vi "Client_Progetto.vi"() -> ()   [LabVIEW 2023]
uses:
  <vilib>/measure/madcrms.llb/Basic Averaged DC-RMS for 1 Chan.vi
  <vilib>/measure/NI_MAPro.lvlib
panel:
  out "Elettromiogramma (EMG)":waveform(dbl)[](graph)
  out "Valore minimo":dbl format="%0.2f"
  out "Valore massimo":dbl format="%0.2f"
  out "Valore efficace (RMS)":dbl format="%0.2p"
  out "error out":errorcluster
  out "error out 2":errorcluster
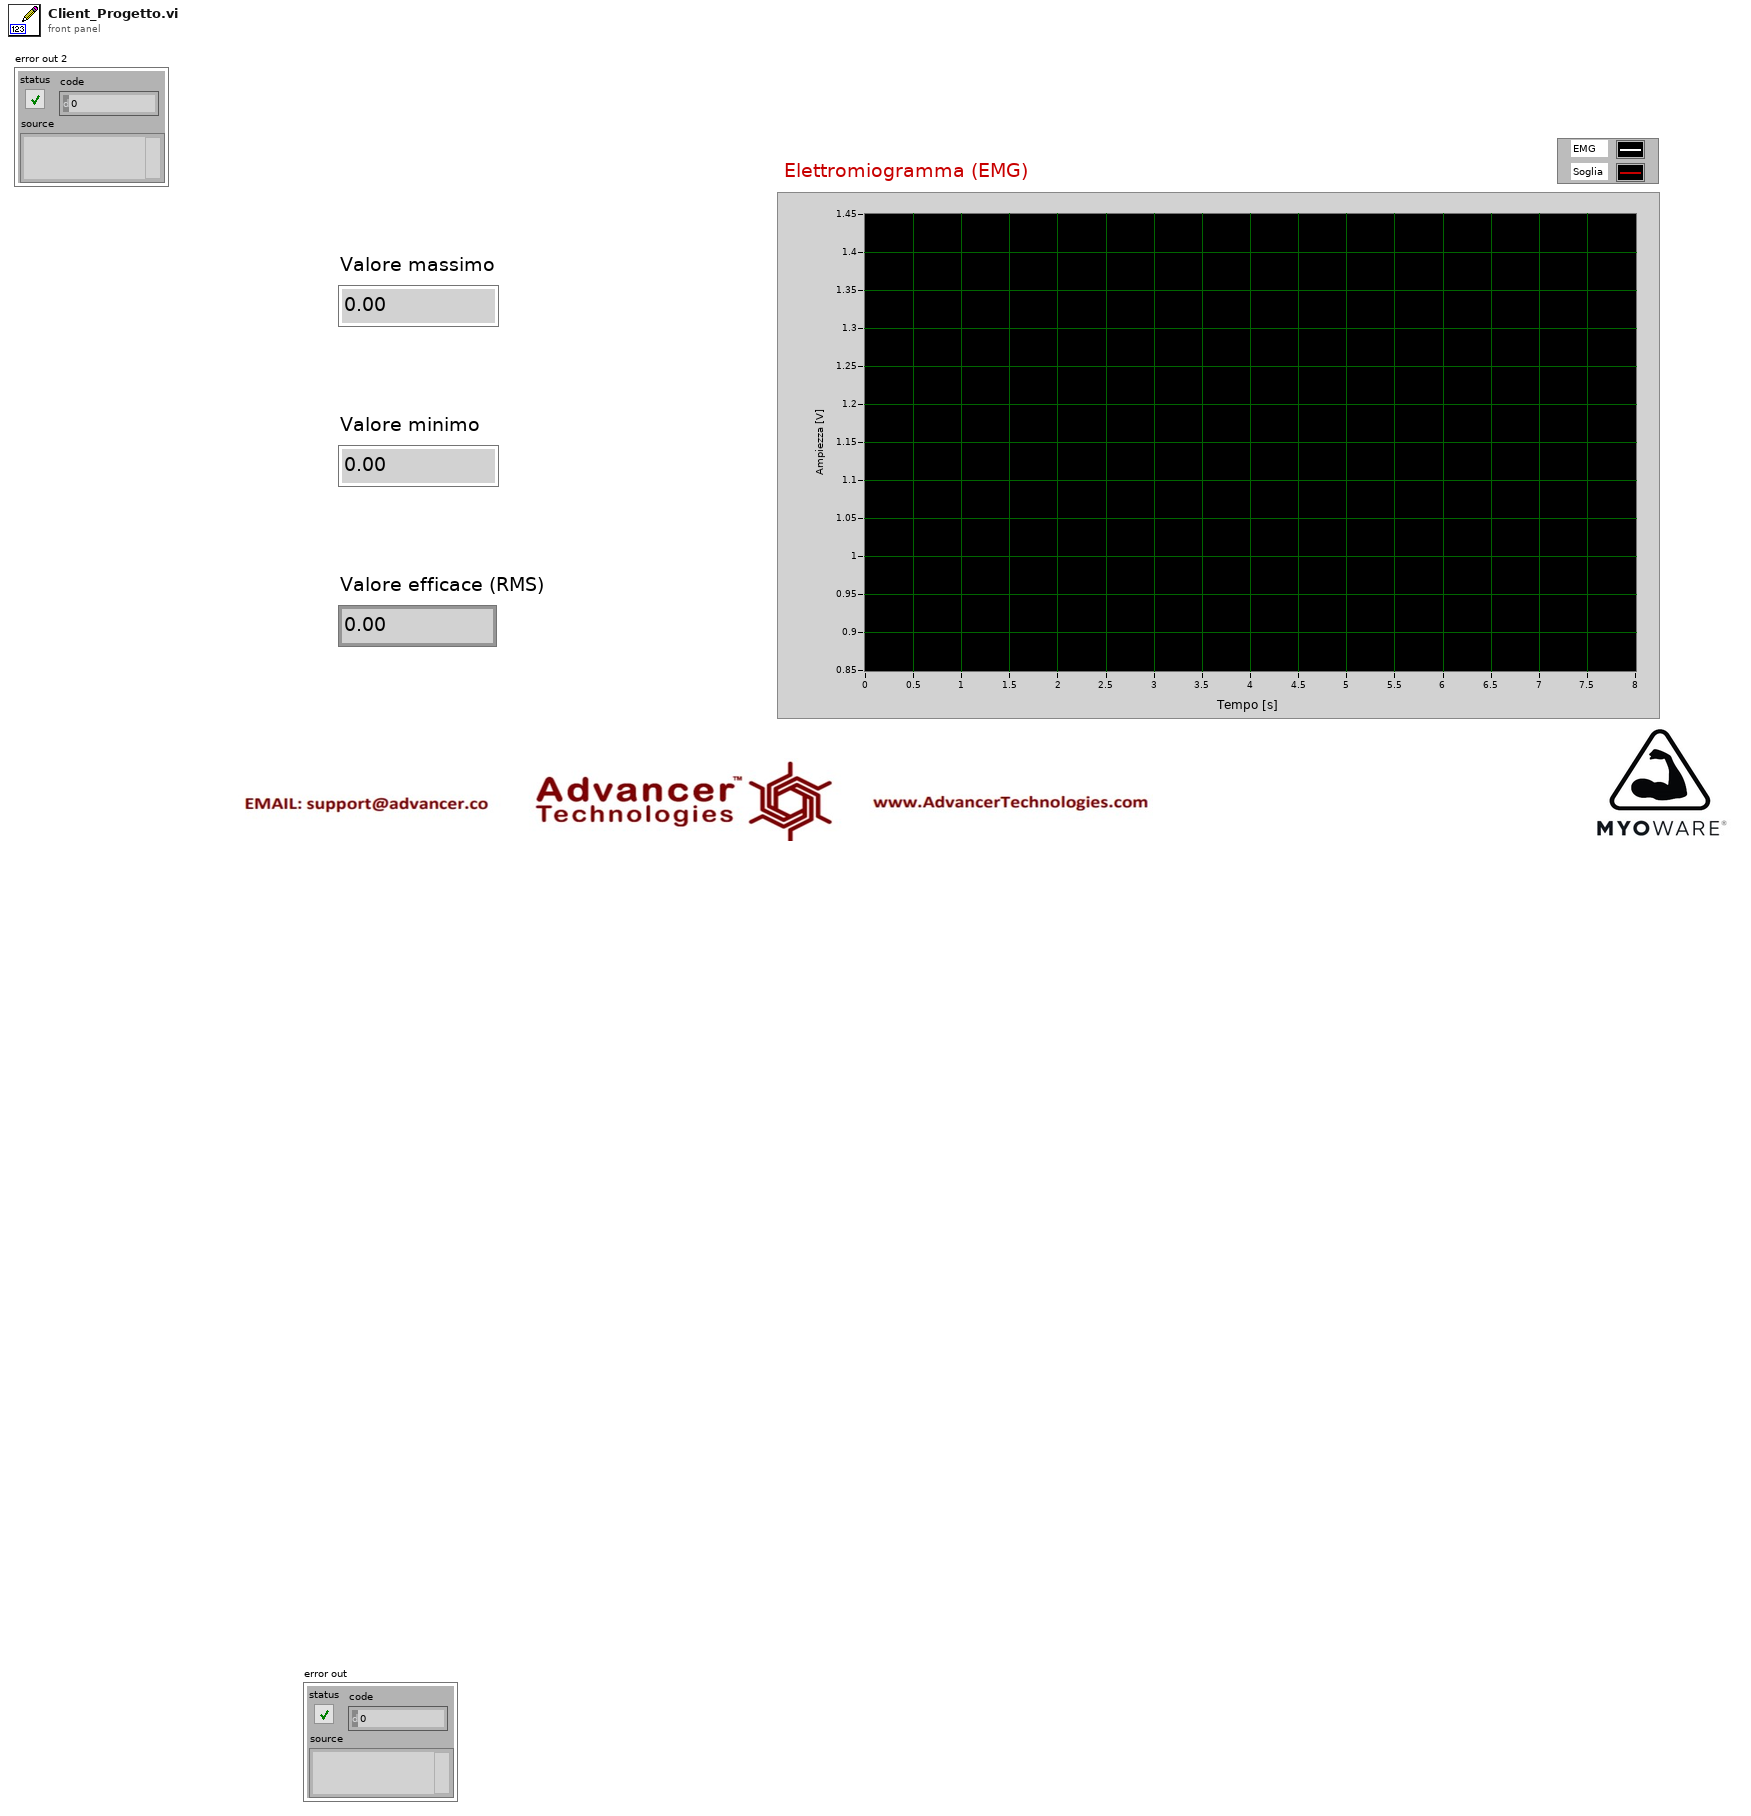
[diagram p1: front panel]
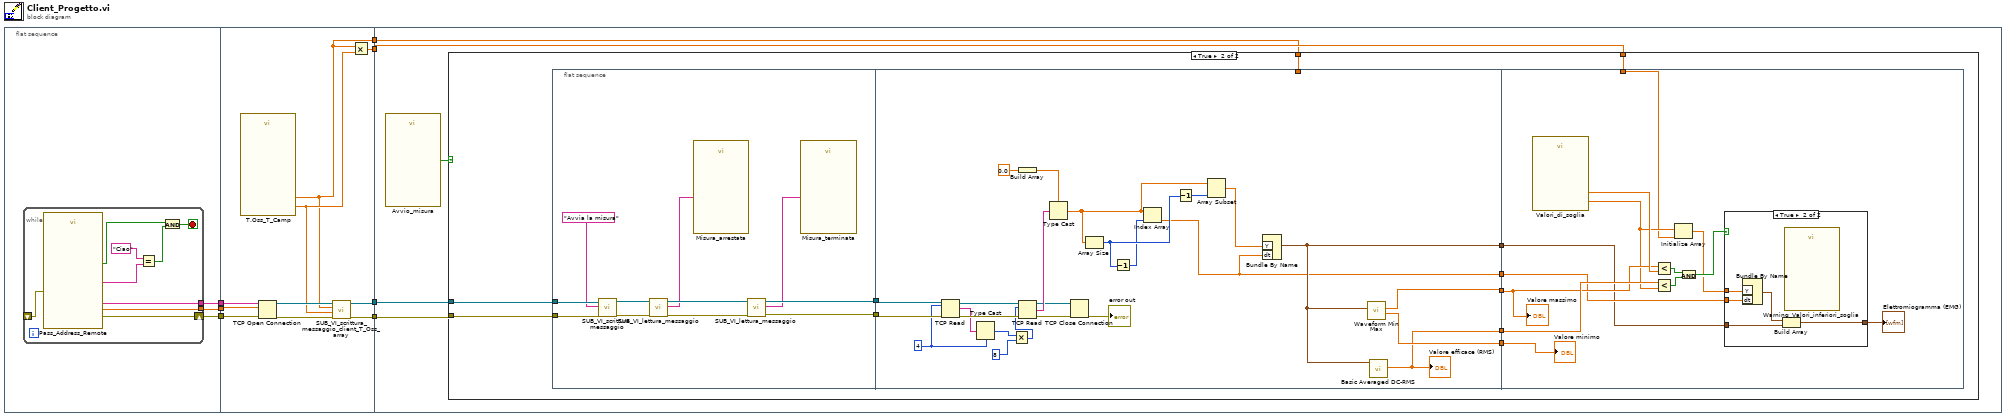
[diagram p0: block diagram]
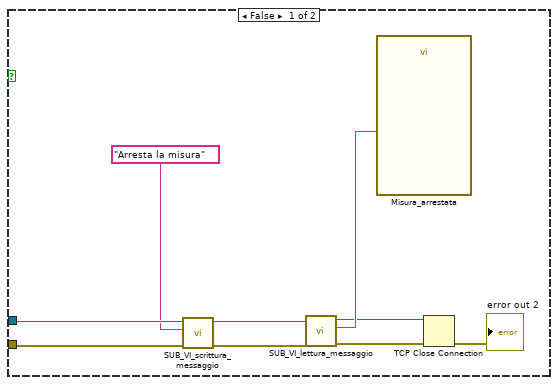
[diagram p2: hidden frame]
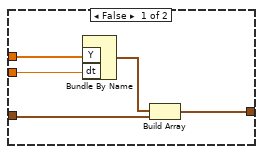
[diagram p3: hidden frame]
diagram:
  n1 = flat-sequence {
    tunnel: [w10] -> w4
    tunnel: [w9] -> w3
    tunnel: [w8] -> w2
    tunnel: [w27] -> w7
    tunnel: [w26] -> w6
    tunnel: [w24] -> w5
    tunnel: w4 -> [w23]
    tunnel: w3 -> [w22]
    tunnel: w2 -> [w21]
    tunnel: [w20] -> w1
    tunnel: w7 -> [w32]
    tunnel: w6 -> [w33]
    tunnel: w5 -> [w31]
    tunnel: w1 -> [w30]
    frame #0 {
      n2 = while {
        shift-right: [w18] -> w8
        shift-left: _ -> [w19]
        tunnel: [w15] -> w10
        tunnel: [w14] -> w9
        stop <- w13 stop-if-true
        n3 = call "Pass_Address_Remote.vi"("error in (no error)"=w19) -> ("Remote port"=w14:dbl, "Address"=w15:string, "Password"=w16:string, "Avanti"=w12:bool, "error out"=w18:errorcluster)  [unwired: 14 in]
        n4 = Equal?(x="Ciao", y=w16) -> (x = y?=w11:bool)
        n5 = And(x=w12, y=w11) -> (x .and. y?=w13:bool)
      }
    }
    frame #1 {
      n6 = call "T.Oss_T_Camp.vi"() -> ("Freq.Campionamento"=w25:dbl, "T.Osservazione"=w20:dbl)  [unwired: 16 in, 2 out]
      n7 = TCP Open Connection(address=w23, remote port or service name=w22, error in (no error)=w21) -> (connection ID=w29:refnum<k5>, error out=w28:errorcluster)  [unwired: 2 in]
      n8 = call "SUB_VI_scrittura_messaggio_client_T_Oss_array.vi"("Errore in ingresso"=w28, "Freq.Campionamento"=w25, "T.Osservazione"=w20, "TCP Network Connection in"=w29) -> ("Errore in uscita"=w27:errorcluster, "TCP Network Connection out"=w26:refnum<k5>)  [unwired: 6 in]
      n9 = Multiply(x=w20, y=w25) -> (x*y=w24:dbl)
    }
    frame #2 {
      n10 = call "Avvio_misura.vi"() -> ("Avviare la misura"=w34:bool)  [unwired: 16 in, 3 out]
      n11 = case shown="True" w34 {
        tunnel: w33 -> [w42 w54]
        tunnel: w32 -> [w41 w53]
        tunnel: w31 -> [_ w46]
        tunnel: w30 -> [_ w44]
        frame False {
          n12 = call "SUB_VI_scrittura_messaggio.vi"("Errore in ingresso"=w41, "Messaggio da inviare"="Arresta la misura", "TCP Network \nConnection in"=w42) -> ("Errore in uscita"=w38:errorcluster, "TCP Network \nConnection out"=w39:refnum<k5>)  [unwired: 7 in]
          n13 = call "SUB_VI_lettura_messaggio.vi"("Errore ingresso"=w38, "TCP Network Connection in"=w39) -> ("Errore uscita"=w36:errorcluster, "Messaggio ricevuto"=w37:string, "TCP Network Connection out"=w35:refnum<k5>)  [unwired: 6 in, 1 out]
          n14 = call "Misura_arrestata.vi"("Message"=w37) -> ()  [unwired: 9 in, 2 out]
          n15 = TCP Close Connection(connection ID=w35, error in (no error)=w36) -> (error out=→"error out 2":errorcluster)  [unwired: 1 in, 1 out]
        }
        frame True {
          n16 = flat-sequence {
            tunnel: w54 -> [w65]
            tunnel: w53 -> [w64]
            tunnel: [w57] -> w52
            tunnel: [w58] -> w51
            tunnel: w52 -> [w73]
            tunnel: w51 -> [w74]
            tunnel: [w72] -> w50
            tunnel: [w71] -> w49
            tunnel: [w70] -> w48
            tunnel: [w67] -> w47
            tunnel: [w69] -> w45
            tunnel: w44 -> [_]
            tunnel: w50 -> [w97]
            tunnel: w49 -> [w99]
            tunnel: w48 -> [w98]
            tunnel: w47 -> [w96]
            tunnel: w46 -> [w94]
            tunnel: w45 -> [w92]
            frame #0 {
              n17 = call "SUB_VI_scrittura_messaggio.vi"("Errore in ingresso"=w64, "Messaggio da inviare"="Avvia la misura", "TCP Network \nConnection in"=w65) -> ("Errore in uscita"=w61:errorcluster, "TCP Network \nConnection out"=w62:refnum<k5>)  [unwired: 7 in]
              n18 = call "SUB_VI_lettura_messaggio.vi"("Errore ingresso"=w61, "TCP Network Connection in"=w62) -> ("Errore uscita"=w59:errorcluster, "Messaggio ricevuto"=w56:string, "TCP Network Connection out"=w60:refnum<k5>)  [unwired: 6 in, 1 out]
              n19 = call "Misura_arrestata.vi"("Message"=w56) -> ()  [unwired: 9 in, 2 out]
              n20 = call "SUB_VI_lettura_messaggio.vi"("Errore ingresso"=w59, "TCP Network Connection in"=w60) -> ("Errore uscita"=w58:errorcluster, "Messaggio ricevuto"=w55:string, "TCP Network Connection out"=w57:refnum<k5>)  [unwired: 6 in, 1 out]
              n21 = call "Misura_terminata.vi"("Message"=w55) -> ()  [unwired: 9 in, 2 out]
            }
            frame #1 {
              w68 = 4 ("bytes to read")
              n22 = TCP Read(connection ID=w73, bytes to read=w68, error in (no error)=w74) -> (connection ID out=w89:refnum<k5>, data out=w84:string, error out=w85:errorcluster)  [unwired: 2 in]
              n23 = Type Cast(type=w68, x=w84) -> (*(type *) &x=w83:i32)
              n24 = Multiply(x=w83, y=8) -> (x*y=w81:i32)
              n25 = Build Array(0.0) -> (w86:dbl[])
              n26 = TCP Read(connection ID=w89, bytes to read=w81, error in (no error)=w85) -> (connection ID out=w76:refnum<k5>, data out=w88:string, error out=w75:errorcluster)  [unwired: 2 in]
              n27 = Type Cast(type=w86, x=w88) -> (*(type *) &x=w80:dbl[])
              n28 = TCP Close Connection(connection ID=w76, error in (no error)=w75) -> (error out=→"error out":errorcluster)  [unwired: 1 in, 1 out]
              n29 = Array Size(array=w80) -> (size(s)=w78:i32)
              n30 = Decrement(x=w78) -> (x-1=w77:i32)
              n31 = Index Array(array=w80, index=w77) -> (element=w67:dbl)
              n32 = Decrement(x=w78) -> (x-1=w79:i32)
              n33 = Array Subset(array=w80, length=w79) -> (w66:dbl[])  [unwired: 1 in]
              n34 = Bundle By Name("Y"=w66, "dt"=w67) -> (w69:waveform(dbl))  [unwired: 1 in]
              n35 = call <vilib>:"Waveform Min Max.vi"("waveform in"=w69) -> ("Y min"=w71:dbl, "Y max"=w72:dbl)  [unwired: 5 in, 4 out]
              n36 = call-poly <vilib>:"Basic Averaged DC-RMS.vi"("signal in"=w69) -> ("RMS value"=w70:dbl)  [unwired: 7 in, 3 out]
              "Valore efficace (RMS)" <- w70
            }
            frame #2 {
              n37 = call "Valori_di_soglia.vi"() -> ("Soglia minima del picco rilevabile"=w95:dbl, "Soglia minima del valore efficace"=w103:dbl)  [unwired: 16 in, 2 out]
              n38 = Less?(x=w97, y=w103) -> (x < y?=w101:bool)
              n39 = Less?(x=w98, y=w95) -> (x < y?=w102:bool)
              n40 = Initialize Array(w95, w94) -> (w93:dbl[])
              n41 = And(x=w101, y=w102) -> (x .and. y?=w100:bool)
              n42 = case shown="True" w100 {
                tunnel: w96 -> [w105 w113]
                tunnel: w93 -> [w107 w112]
                tunnel: w92 -> [w106 w110]
                tunnel: [w104 w109] -> w91
                frame False {
                  n43 = Bundle By Name("Y"=w107, "dt"=w105) -> (w108:waveform(dbl))  [unwired: 1 in]
                  n44 = Build Array(w106, w108) -> (w104:waveform(dbl)[])
                }
                frame True {
                  n45 = Bundle By Name("Y"=w112, "dt"=w113) -> (w111:waveform(dbl))  [unwired: 1 in]
                  n46 = Build Array(w111, w110) -> (w109:waveform(dbl)[])
                  n47 = call "Warning_Valori_inferiori_soglia.vi"() -> ()  [unwired: 10 in, 2 out]
                }
              }
              "Elettromiogramma (EMG)" <- w91
              "Valore massimo" <- w97
              "Valore minimo" <- w99
            }
          }
        }
      }
    }
  }
